vi "SimpleCurveAdded Event Callback.vi"(4 "User Parameter":T1, 5 "Event Data":T2, 6 "Control Ref":refnum<k24>, 7 "Event Common Data":T3) -> ()   [LabVIEW 2020]
uses:
  C:/Utils/LabVIEWNETSDK - Class/PalmSens/Libraries/PalmSens.Core.Simplified.dll
  Libraries/PalmSens.Core.Simplified.dll
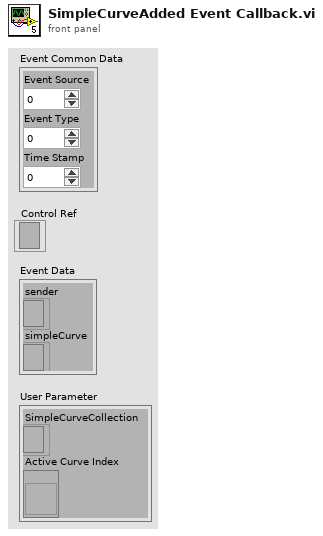
[diagram p1: front panel]
types:
  T1 = cluster{"SimpleCurveCollection":refnum<k24>, "Active Curve Index":refnum<vi>}
  T2 = cluster{"sender":refnum<k24>, "simpleCurve":refnum<k24>}
  T3 = cluster{"Event Source":i32, "Event Type":u32, "Time Stamp":u32}
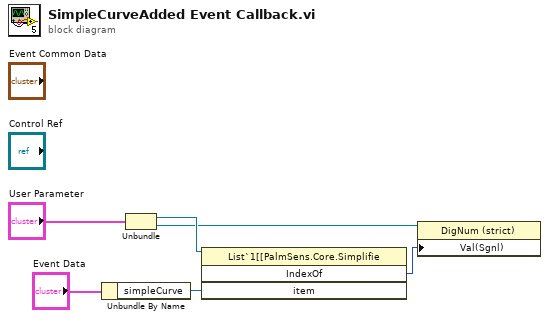
[diagram p0: block diagram]
diagram:
  n1 = Unbundle By Name("Event Data") -> ("simpleCurve"=w3:refnum<k24>)
  n2 = Unbundle("User Parameter") -> ("SimpleCurveCollection"=w5:refnum<k24>, "Active Curve Index"=w2:refnum<vi>)
  n3 = invoke class="List`1[[PalmSens.Core.Simplifie" method="IndexOf"(reference=w5, "item"=w3) -> ("IndexOf"=w1:i32)  [unwired: 2 in, 3 out]
  n4 = property class="DigNum (strict)"(reference=w2, "Val(Sgnl)"=w1) -> ()  [unwired: 1 in, 2 out]
